vi "Cross Entropy.vi"(9 "Q(x)":dbl[][][](array[numeric])=[[[0.20328533], [0.10445738], [0.69225729]], [[0.24201603], [0.17203346], [0.58595051]]] format="%_8f", 11 "P(x)":dbl[][][](array[numeric])=[[[1.0], [0.0], [0.0]], [[0.0], [1.0], [0.0]]]) -> (1 "Cross Entropy (Array)":dbl[](array[numeric])=[1.5931447203218374, 1.7600662862044198] format="%_8f", 3 "Cross Entropy (total)":dbl=3.3532110065262573 format="%_8f")   [LabVIEW 2014]
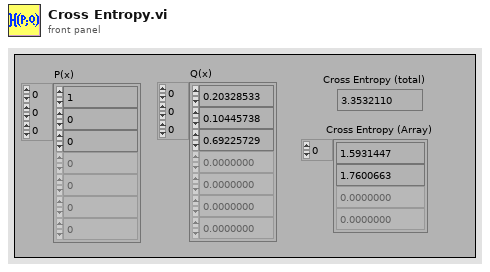
[diagram p1: front panel]
types:
  T1 = typedef "NI_Matrix.lvlib/RealMatrix.ctl" = dbl[][]
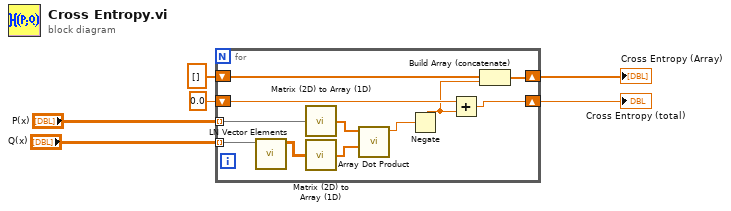
[diagram p0: block diagram]
diagram:
  n1 = for {
    tunnel: "P(x)" -> [w11] mode=indexing
    shift-right: [w16] -> w5
    shift-left: 0.0 -> [w17]
    shift-right: [w7] -> w6
    shift-left: dbl[] [] -> [w15]
    tunnel: "Q(x)" -> [w14] mode=indexing
    n2 = call "LN Vector Elements.vi"("Vector (in)"=w14) -> ("Real Matrix (Column Vector)"=w13:T1)  [unwired: 10 in]
    n3 = call "Matrix (2D) to Array (1D).vi"("Matrix (2D)"=w11) -> ("Array (1D)"=w10:dbl[])  [unwired: 4 in]
    n4 = call "Matrix (2D) to Array (1D).vi"("Matrix (2D)"=w13) -> ("Array (1D)"=w12:dbl[])  [unwired: 4 in]
    n5 = call "Array Dot Product.vi"("array a"=w10, "array b"=w12) -> ("a . b"=w9:dbl)  [unwired: 8 in]
    n6 = Negate(x=w9) -> (-x=w8:dbl)
    n7 = Add(x=w17, y=w8) -> (x+y=w16:dbl)
    n8 = Build Array (concatenate)(w15, w8) -> (w7:dbl[])
  }
  "Cross Entropy (Array)" <- w6
  "Cross Entropy (total)" <- w5
